vi "Get Message Type.vi"(8 "error in (no error)":errorcluster, 11 "SECS-II Class in":refnum<class "SECS-II Class.lvclass">) -> (0 "error out":errorcluster, 1 "Reply?":bool, 2 "Message Type":string, 3 "SECS-II Class out":refnum<class "SECS-II Class.lvclass">)   [LabVIEW 2020, in "SECS Communication.lvlib" / "SECS-II Class.lvclass"]
uses:
  SECS-II Class.lvclass
  SECS-II Class.lvclass/SECS-II Class.ctl
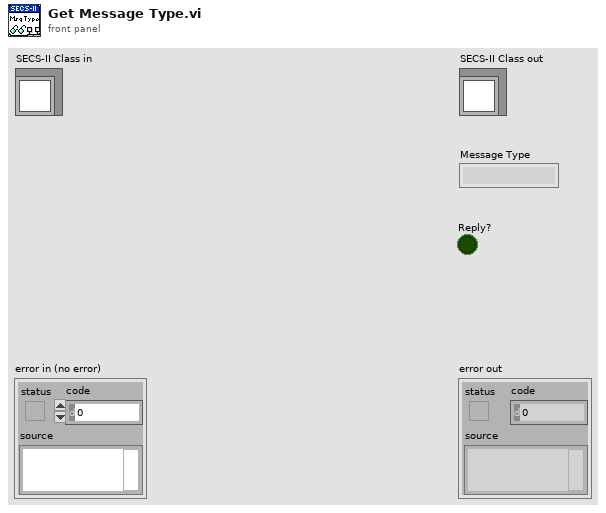
[diagram p1: front panel]
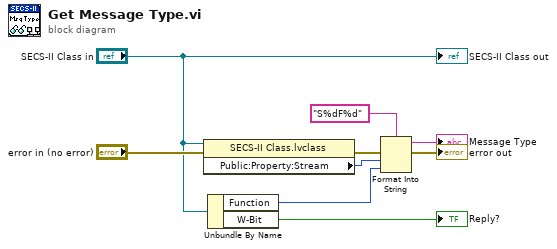
[diagram p0: block diagram]
diagram:
  n1 = property class="SECS-II Class.lvclass"(reference="SECS-II Class in", error in="error in (no error)") -> (error out=w7:errorcluster, "Public:Property:Stream"=w6:u8)  [unwired: 1 out]
  n2 = Unbundle By Name("SECS-II Class in") -> ("Function"=w5:u8, "W-Bit"=→"Reply?":bool)
  n3 = Format Into String(format string="S%dF%d", error in=w7, w6, w5) -> (resulting string=→"Message Type":string, error out=→"error out":errorcluster)  [unwired: 1 in]
  "SECS-II Class out" <- "SECS-II Class in"
